vi "Populate.vi"(8 "error in (no error)":errorcluster, 9 "Display Text Array":string[](array[string]), 10 "Values Array":variant, 11 "Ring Ctrl Value Source in":refnum<class "Ring Ctrl Value Source.lvclass">) -> (0 "error out":errorcluster, 3 "Ring Ctrl Value Source out":refnum<class "Ring Ctrl Value Source.lvclass">)   [LabVIEW 2020, in "Composed Columns.lvlib" / "Ring Ctrl Value Source.lvclass"]
uses:
  Ring Ctrl Value Source.lvclass
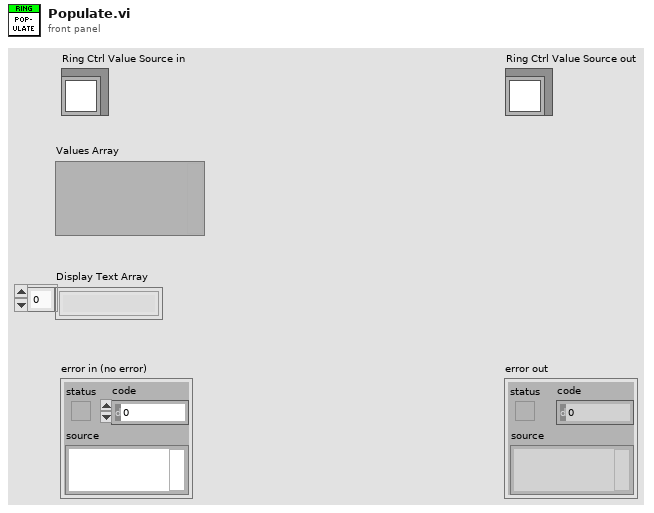
[diagram p1: front panel]
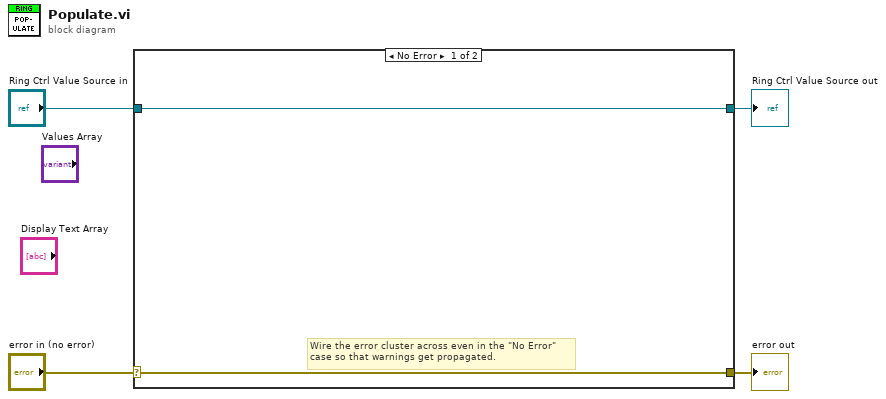
[diagram p0: block diagram]
diagram:
  n1 = case shown="No Error" "error in (no error)" {
    selector: "error in (no error)" -> [w5 w8]
    tunnel: [w5 w8] -> w3
    tunnel: [w6 w7] -> w1
    tunnel: "Ring Ctrl Value Source in" -> [w6 w7]
    frame No Error {
      # "Wire the error cluster across even in the \"No Error\"\ncase so that warnings get propagated."
    }
    frame Error {
    }
  }
  "error out" <- w3
  "Ring Ctrl Value Source out" <- w1
